vi "FTW-Logger-Process.vi"(0 "FTW Logger Configuration":string, 11 "error in":errorcluster) -> (15 "error out":errorcluster)   [LabVIEW 2013, in "FTW-Logger-Instance.lvclass"]
uses:
  FTW-Logger-Instance.lvclass
  FTW-Logger.lvclass
  instance/FTW-Actor-Instance.lvclass
  request/FTW-Request.lvclass
panel:
  # "Inputs"
  # "Outputs"
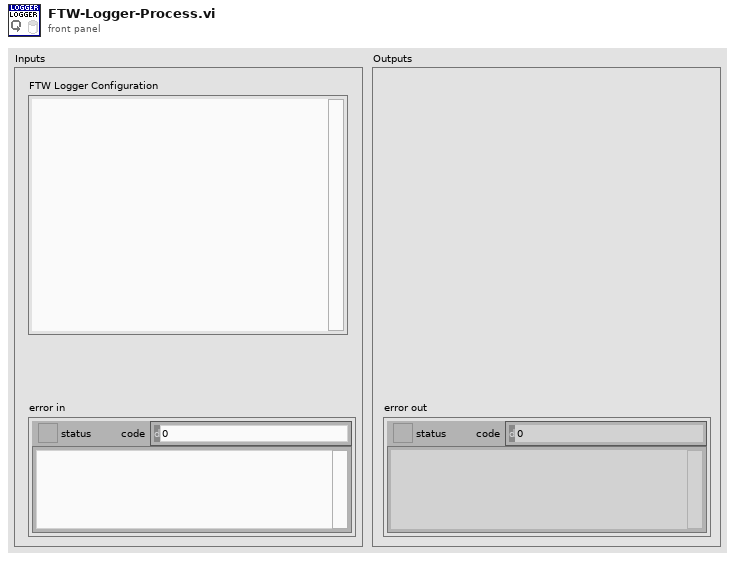
[diagram p1: front panel]
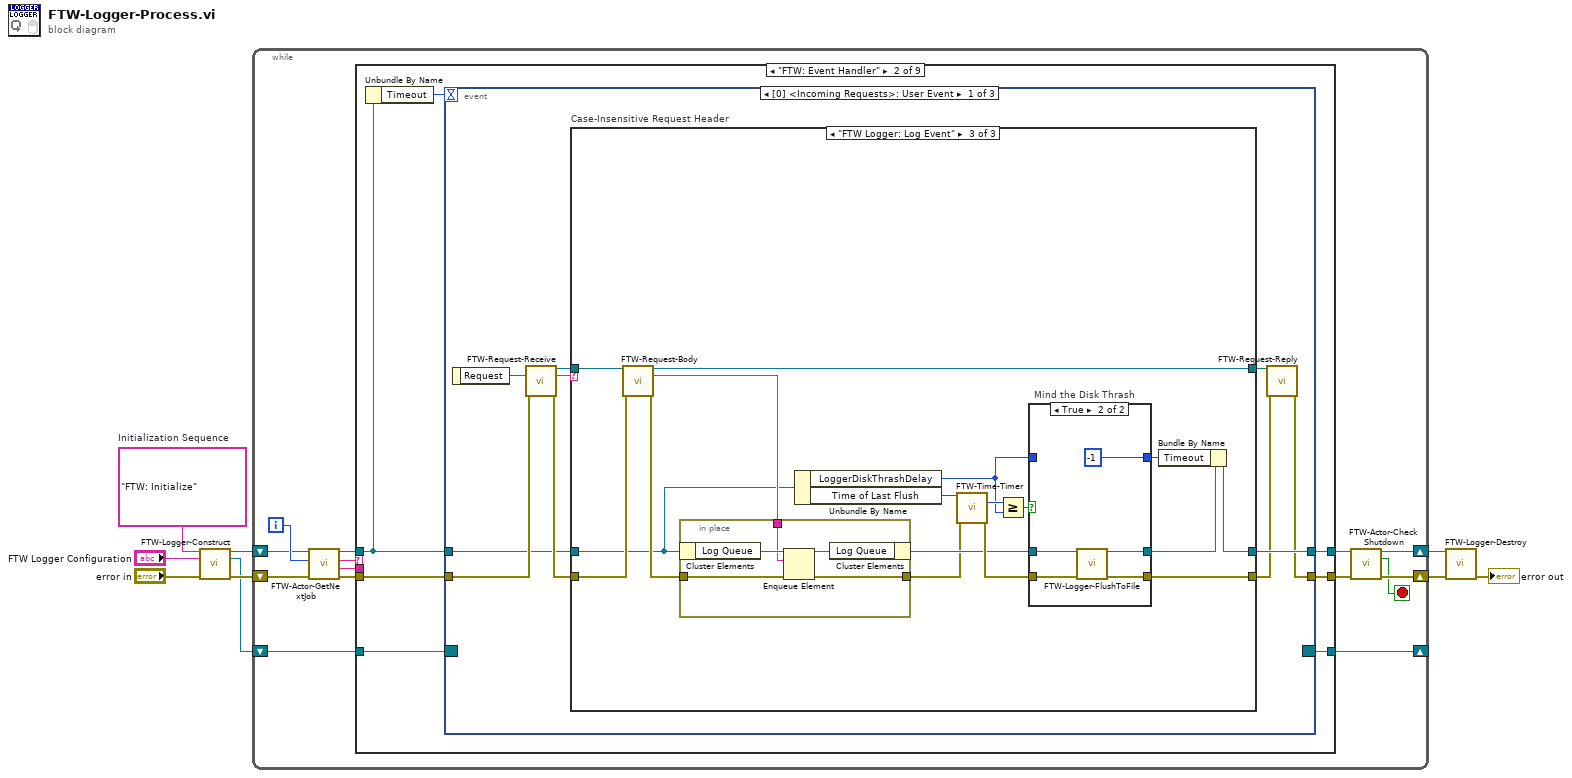
[diagram p0: block diagram]
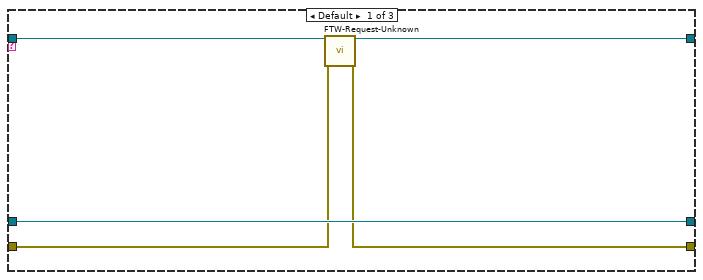
[diagram p3: hidden frame]
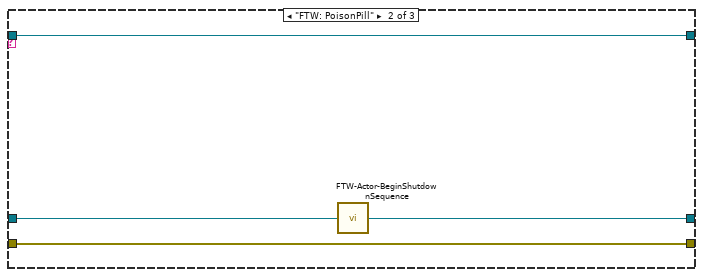
[diagram p4: hidden frame]
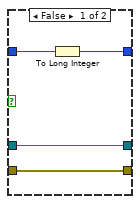
[diagram p5: hidden frame]
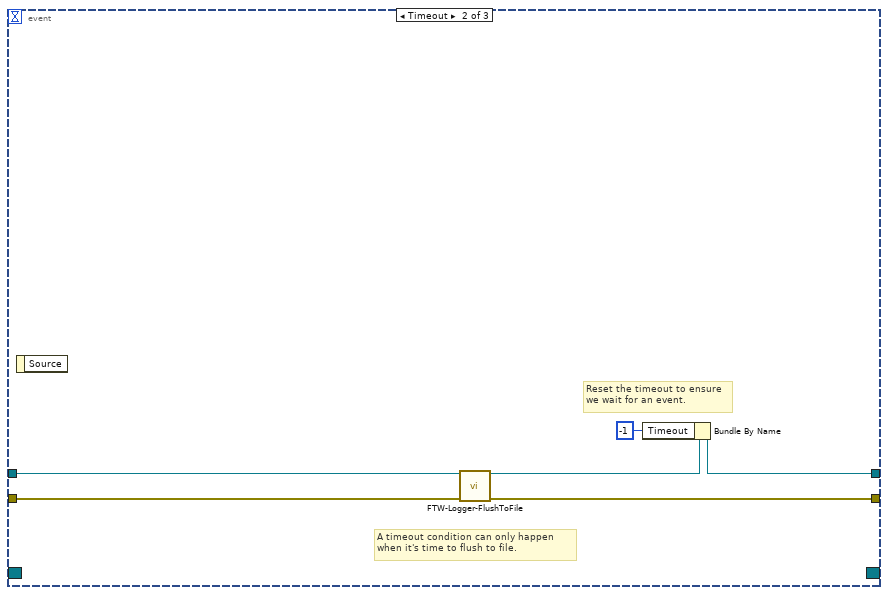
[diagram p6: hidden frame]
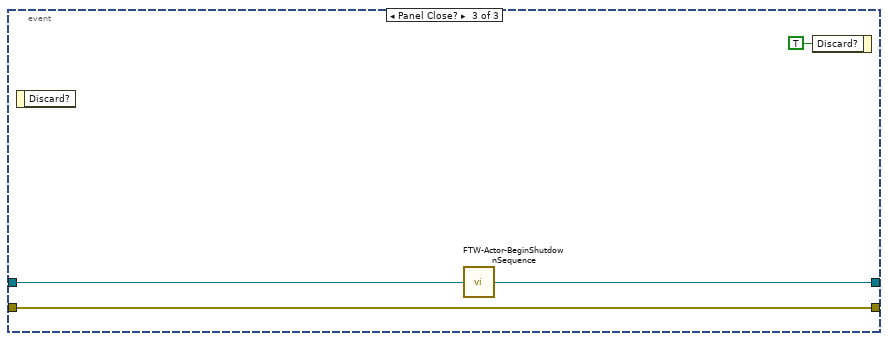
[diagram p7: hidden frame]
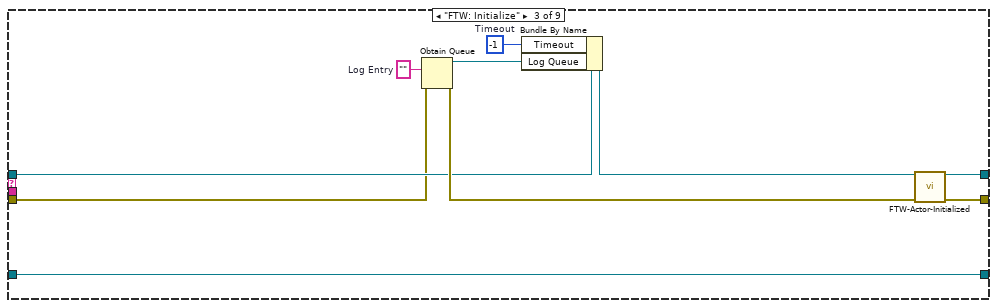
[diagram p8: hidden frame]
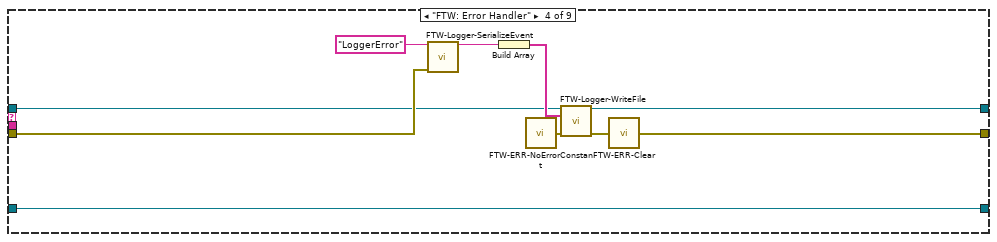
[diagram p9: hidden frame]
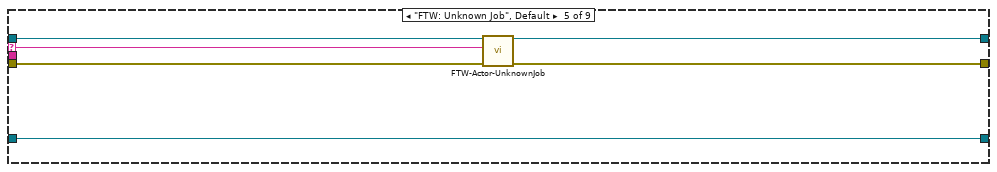
[diagram p10: hidden frame]
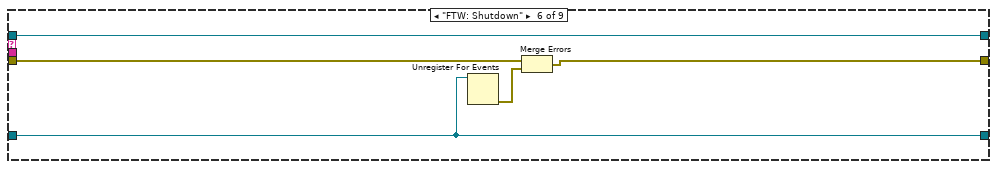
[diagram p11: hidden frame]
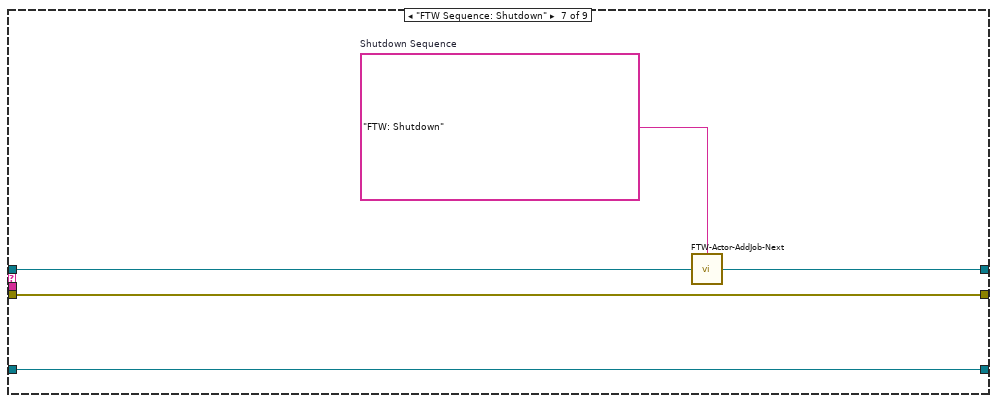
[diagram p12: hidden frame]
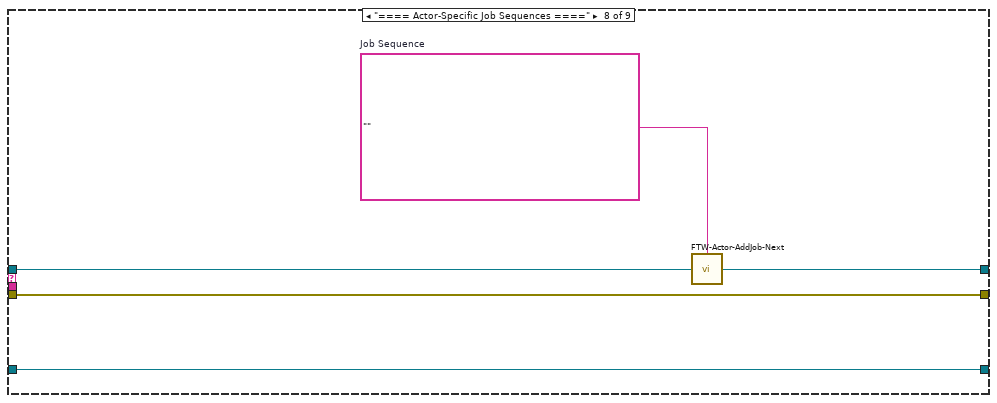
[diagram p13: hidden frame]
diagram:
  w2 = "FTW: Initialize"  # Initialization Sequence
  n1 = call "FTW-Logger-Construct.vi"("Initialization Sequence"=w2, "Logger Configuration"="FTW Logger Configuration", "error in"="error in") -> ("FTW Logger"=w6:refnum<class "FTW-Logger-Instance.lvclass">, "Incoming Requests"=w3:refnum<event-registration>, "error out"=w5:errorcluster)  [unwired: 10 in]
  n2 = while {
    shift-right: [w12] -> w8
    shift-left: w5 -> [w21]
    shift-right: [w22] -> _
    shift-left: w3 -> [w23]
    shift-right: [w11] -> w9
    shift-left: w6 -> [w18]
    i -> [w20]
    stop <- w10 stop-if-true
    n3 = call "FTW-Actor-GetNextJob.vi"("error in"=w21, "Jobs Performed"=w20, "FTW Actor Instance"=w18) -> ("error out"=w19:errorcluster, "Job Data"=w15:string, "Job Name"=w16:string, "FTW Actor Instance out"=w17:refnum<class "FTW-Logger-Instance.lvclass">)  [unwired: 5 in]
    n4 = case shown="\"FTW: Event Handler\"" w16 {
      selector: w16 -> [_ _ _ _ w115 _ _ _ _]
      tunnel: [w25 w33 w99 w109 w116 w124 w128 w133 w137] -> w13
      tunnel: w19 -> [w25 w32 w94 w111 w114 w120 w128 w133 w137]
      tunnel: w23 -> [w26 w31 w102 w113 w119 w122 w129 w134 w136]
      tunnel: [w26 w30 w102 w113 w119 w122 w129 w134 w136] -> w22
      tunnel: w17 -> [w24 w27 w95 w105 w118 w121 w126 w131 w135]
      tunnel: [w24 w28 w100 w106 w117 w121 w125 w130 w135] -> w14
      tunnel: w15 -> [_ _ _ _ _ _ _ _ _]
      frame "==== Featherweight Framework Jobs ====" {
      }
      frame "FTW: Event Handler" {
        n5 = Unbundle By Name(w27) -> ("Timeout"=w29:i32)
        n6 = event shown="[0] <Incoming Requests>: User Event" {
          selector: w31 -> [_ _ _]
          dyn-events: [_ _ _] -> w30
          timeout: w29 -> [_ _ _]
          tunnel: [w36 w88 w92] -> w33
          tunnel: w32 -> [w42 w89 w92]
          tunnel: [w41 w84 w90] -> w28
          tunnel: w27 -> [w40 w87 w91]
          event User Event {
            n7 = event-data() -> ("Request"=w34:refnum<class "FTW-Message.lvclass">)  [unwired: 1 in]
            n8 = call "FTW-Request-Receive.vi"("Incoming Message (expected type is Request)"=w34, "error in"=w42) -> ("Initialized Request"=w38:refnum<class "FTW-Request.lvclass">, "Request Header"=w39:string, "error out"=w43:errorcluster)  [unwired: 11 in]
            n9 = case "Case-Insensitive Request Header" shown="\"FTW Logger: Log Event\"" w39 {
              tunnel: [w45 w52 w66] -> w35
              tunnel: w43 -> [w46 w52 w55]
              tunnel: [w48 w50 w62] -> w41
              tunnel: w40 -> [w48 w51 w53]
              tunnel: w38 -> [w47 w49 w58]
              tunnel: [w44 w49 w57] -> w37
              frame Default {
                n10 = call "FTW-Request-Unknown.vi"("FTW Incoming Request"=w47, "error in"=w46) -> ("FTW Incoming Request out"=w44:refnum<class "FTW-Request.lvclass">, "error out"=w45:errorcluster)  [unwired: 12 in]
              }
              frame "FTW: PoisonPill" {
                n11 = call "FTW-Actor-BeginShutdownSequence.vi"("FTW Actor Instance"=w51) -> ("FTW Actor Instance out"=w50:refnum<class "FTW-Logger-Instance.lvclass">)  [unwired: 3 in]
              }
              frame "FTW Logger: Log Event" {
                n12 = call "FTW-Request-Body.vi"("FTW Request"=w58, "error in"=w55) -> ("FTW Request out"=w57:refnum<class "FTW-Request.lvclass">, "Request Body"=w56:string, "error out"=w54:errorcluster)  [unwired: 11 in]
                n13 = in-place {
                  in-place-border: w54 -> [w74]
                  in-place-border: [w71] -> w60
                  in-place-border: w56 -> [w70]
                  n14 = in-place-cluster #1(w53) -> ("Log Queue"=w73:refnum<queue>)
                  n15 = Enqueue Element(queue=w73, element=w70, error in (no error)=w74) -> (queue out=w72:refnum<queue>, error out=w71:errorcluster)  [unwired: 1 in, 1 out]
                  n16 = in-place-cluster #1("Log Queue"=w72) -> (w61:refnum<class "FTW-Logger-Instance.lvclass">)
                }
                n17 = Unbundle By Name(w53) -> ("LoggerDiskThrashDelay"=w59:u32, "Time of Last Flush"=w69:u32)
                n18 = call "FTW-Time-Timer.vi"("Initial Tick Count"=w69, "error in"=w60) -> ("Elapsed Time"=w68:u32, "error out"=w67:errorcluster)  [unwired: 11 in, 1 out]
                n19 = Greater Or Equal?(x=w68, y=w59) -> (x >= y?=w65:bool)
                n20 = case "Mind the Disk Thrash" shown="True" w65 {
                  tunnel: [w78 w80] -> w63
                  tunnel: w61 -> [w78 w81]
                  tunnel: w67 -> [w77 w83]
                  tunnel: [w77 w82] -> w66
                  tunnel: [w75 -1 ("Timeout")] -> w64
                  tunnel: w59 -> [w76 _]
                  frame False {
                    n21 = To Long Integer(number=w76) -> (32bit integer=w75:i32)
                  }
                  frame True {
                    n22 = call "FTW-Logger-FlushToFile.vi"("FTW Logger"=w81, "error in"=w83) -> ("FTW Logger out"=w80:refnum<class "FTW-Logger-Instance.lvclass">, "error out"=w82:errorcluster)  [unwired: 12 in]
                  }
                }
                n23 = Bundle By Name(cluster=w63, "Timeout"=w64) -> (w62:refnum<class "FTW-Logger-Instance.lvclass">)
              }
            }
            n24 = call "FTW-Request-Reply.vi"("FTW Incoming Request"=w37, "error in"=w35) -> ("error out"=w36:errorcluster)  [unwired: 12 in, 1 out]
          }
          event Timeout {
            # "Reset the timeout to ensure\nwe wait for an event."
            # "A timeout condition can only happen\nwhen it's time to flush to file."
            n25 = event-data() -> ()  [unwired: 1 in, 1 out]
            n26 = call "FTW-Logger-FlushToFile.vi"("FTW Logger"=w87, "error in"=w89) -> ("FTW Logger out"=w85:refnum<class "FTW-Logger-Instance.lvclass">, "error out"=w88:errorcluster)  [unwired: 12 in]
            n27 = Bundle By Name(cluster=w85, "Timeout"=-1) -> (w84:refnum<class "FTW-Logger-Instance.lvclass">)
          }
          event Panel Close? {
            n28 = event-data() -> ()  [unwired: 1 in, 1 out]
            n29 = call "FTW-Actor-BeginShutdownSequence.vi"("FTW Actor Instance"=w91) -> ("FTW Actor Instance out"=w90:refnum<class "FTW-Logger-Instance.lvclass">)  [unwired: 3 in]
            n30 = event-data("Discard?"=TRUE) -> ()  [unwired: 1 in, 1 out]
          }
        }
      }
      frame "FTW: Initialize" {
        w96 = ""  # Log Entry
        w103 = -1  # Timeout
        n31 = Obtain Queue(element data type=w96, error in (no error)=w94) -> (queue out=w98:refnum<queue>, error out=w97:errorcluster)  [unwired: 3 in, 1 out]
        n32 = Bundle By Name(cluster=w95, "Timeout"=w103, "Log Queue"=w98) -> (w101:refnum<class "FTW-Logger-Instance.lvclass">)
        n33 = call-dynamic "FTW-Actor-Initialized.vi"("FTW Actor Instance"=w101, "error in"=w97) -> ("FTW Actor Instance out"=w100:refnum<class "FTW-Logger-Instance.lvclass">, "error out"=w99:errorcluster)  [unwired: 12 in]
      }
      frame "FTW: Error Handler" {
        n34 = call "FTW-Logger-SerializeEvent.vi"("Event Type"="LoggerError", "Error to Log"=w111) -> ("Serialized Event"=w108:string)  [unwired: 13 in]
        n35 = Build Array(w108) -> (w107:string[])
        n36 = call "FTW-ERR-NoErrorConstant.vi"() -> ("no error"=w104:errorcluster)
        n37 = call "FTW-Logger-WriteFile.vi"("FTW Logger"=w105, "Entries to Log"=w107, "error in"=w104) -> ("FTW Logger out"=w106:refnum<class "FTW-Logger-Instance.lvclass">, "error out"=w110:errorcluster)  [unwired: 11 in]
        n38 = call "FTW-ERR-Clear.vi"("error to snuff"=w110) -> ("no error"=w109:errorcluster)
      }
      frame "FTW: Unknown Job", Default {
        n39 = call-dynamic "FTW-Actor-UnknownJob.vi"("FTW Actor Instance"=w118, "Unknown Job"=w115, "error in"=w114) -> ("FTW Actor Instance out"=w117:refnum<class "FTW-Logger-Instance.lvclass">, "error out"=w116:errorcluster)  [unwired: 11 in]
      }
      frame "FTW: Shutdown" {
        n40 = Unregister For Events(event registration refnum=w122) -> (error out=w123:errorcluster)  [unwired: 1 in]
        n41 = Merge Errors(w120, w123) -> (w124:errorcluster)
      }
      frame "FTW Sequence: Shutdown" {
        w127 = "FTW: Shutdown"  # Shutdown Sequence
        n42 = call "FTW-Actor-AddJob-Next.vi"("Add Next in Job Queue"=w127, "FTW Actor Instance"=w126) -> ("FTW Actor Instance out"=w125:refnum<class "FTW-Logger-Instance.lvclass">)  [unwired: 2 in]
      }
      frame "==== Actor-Specific Job Sequences ====" {
        w132 = ""  # Job Sequence
        n43 = call "FTW-Actor-AddJob-Next.vi"("Add Next in Job Queue"=w132, "FTW Actor Instance"=w131) -> ("FTW Actor Instance out"=w130:refnum<class "FTW-Logger-Instance.lvclass">)  [unwired: 2 in]
      }
      frame "==== Actor-Specific Jobs ====" {
      }
    }
    n44 = call "FTW-Actor-CheckShutdown.vi"("FTW Actor Instance"=w14, "error in"=w13) -> ("FTW Actor Instance out"=w11:refnum<class "FTW-Logger-Instance.lvclass">, "Shutdown?"=w10:bool, "error out"=w12:errorcluster)  [unwired: 11 in]
  }
  n45 = call "FTW-Logger-Destroy.vi"("FTW Logger"=w9, "error in"=w8) -> ("error out"=→"error out":errorcluster)  [unwired: 13 in]
